vi "Read PhysChan.Properties.vi"(8 "error in (no error)":errorcluster, 11 "SLSC Local in":refnum<class "SLSC Local.lvclass">) -> (0 "error out":errorcluster, 2 "PhysChan.Properties":refnum<k21>[](array[refnum]), 3 "SLSC Local out":refnum<class "SLSC Local.lvclass">)   [LabVIEW 2015, in "SLSC Local.lvclass"]
uses:
  SLSC Local.lvclass
  SLSC Interface Class/SLSC Interface.lvclass
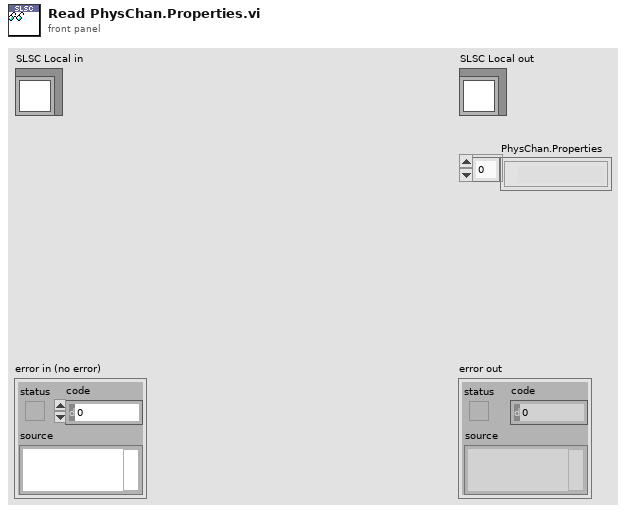
[diagram p1: front panel]
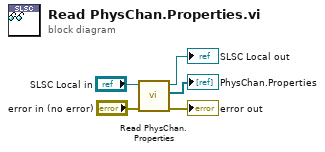
[diagram p0: block diagram]
diagram:
  n1 = call-parent "Read PhysChan.Properties.vi"("error in (no error)"="error in (no error)", "SLSC Interface in"="SLSC Local in") -> ("error out"=→"error out":errorcluster, "PhysChan.Properties"=→"PhysChan.Properties":refnum<k21>[], "SLSC Interface out"=→"SLSC Local out":refnum<class "SLSC Local.lvclass">)  [unwired: 7 in]
